vi "Save Orientation History.vi"() -> (2 "File Name refnum":refnum<file>, 3 "File Name path":path)   [LabVIEW 2016]
uses:
  navxmxp/roborio/labviewae/_TypeDefs/FRIC_navX_DeviceNumbersTypeDef.ctl
  <vilib>/Utility/file.llb/Write Delimited Spreadsheet (DBL).vi
panel:
  out "iterations":i32
  in  "Device Number":T1
  out "error out":errorcluster
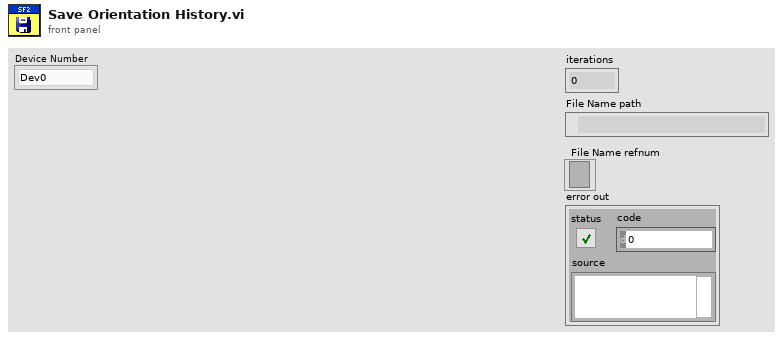
[diagram p1: front panel]
types:
  T1 = typedef "FRIC_navX_DeviceNumbersTypeDef.ctl" = enum16{"Dev0", "Dev1", "Dev2", "Dev3"}
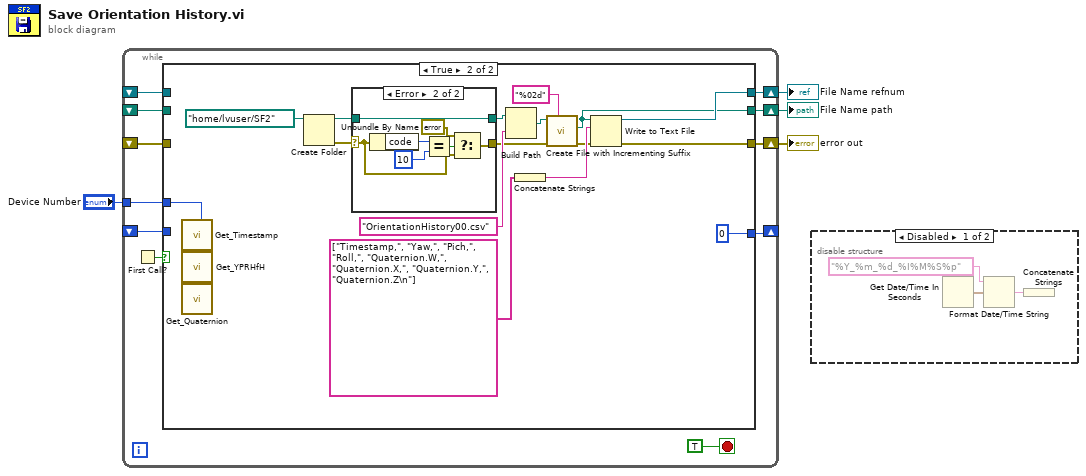
[diagram p0: block diagram]
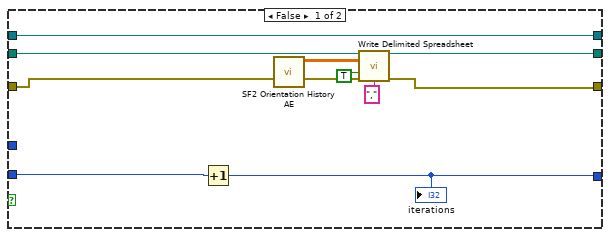
[diagram p3: hidden frame]
diagram:
  n1 = while {
    shift-right: [w15] -> w4
    shift-left: _ -> [w11]
    shift-right: [w14] -> w1
    shift-left: _ -> [w10]
    shift-right: [w9] -> w3
    shift-left: _ -> [w8]
    tunnel: "Device Number" -> [w7]
    shift-right: [w6] -> _
    shift-left: _ -> [w5]
    stop <- TRUE stop-if-true
    n2 = First Call?() -> (First Call?: T/F=w12:bool)
    n3 = case shown="True" w12 {
      tunnel: [w23 w38] -> w15
      tunnel: [w22 w37] -> w14
      tunnel: w11 -> [w23 _]
      tunnel: w10 -> [w21 _]
      tunnel: [w24 w26] -> w9
      tunnel: w8 -> [w25 _]
      tunnel: w7 -> [_ w33]
      tunnel: [w16 0] -> w6
      tunnel: w5 -> [w17 _]
      frame False {
        n4 = Increment(x=w17) -> (x+1=w16:i32)
        "iterations" <- w16
        n5 = call "SF2 Orientation History AE.vi"() -> ("SF2 Buffer (out)"=w18:dbl[][])  [unwired: 10 in, 1 out]
        n6 = call-poly <vilib>:"Write Delimited Spreadsheet.vi"("file path (dialog if empty)"=w25, "2D data"=w18, "append to file? (new file:F)"=TRUE, "error in (no error)"=w21, "delimiter (\\t)"="," ("delimiter (\\t)")) -> ("new file path (Not A Path if cancelled)"=w24:path, "error out"=w22:errorcluster)  [unwired: 9 in]
      }
      frame True {
        n7 = call "Get_Timestamp.vi"("Device Number"=w33) -> ()  [unwired: 10 in, 1 out]
        n8 = call "Get_YPRHfH.vi"("Device Number"=w33) -> ()  [unwired: 10 in, 1 out]
        n9 = call "Get_Quaternion.vi"("Device Number"=w33) -> ()  [unwired: 10 in, 1 out]
        n10 = Create Folder(path (use dialog)=path "/home/lvuser/SF2") -> (created path=w34:path, error out=w36:errorcluster)  [unwired: 2 in, 1 out]
        n11 = case shown="Error" w36 {
          selector: w36 -> [w42 w46]
          tunnel: w34 -> [w43 w50]
          tunnel: [w43 w50] -> w35
          tunnel: [w42 w45] -> w28
          frame No Error {
          }
          frame Error {
            n12 = Unbundle By Name(w46) -> ("code"=w49:i32)
            n13 = Equal?(x=w49, y=10) -> (x = y?=w44:bool)
            n14 = Select(t=errorcluster {"status"=FALSE, "code"=0, "source"=""} ("error IO"), s=w44, f=w46) -> (s? t:f=w45:errorcluster)
          }
        }
        n15 = Build Path(base path=w35, name or relative path="OrientationHistory00.csv") -> (appended path=w30:path)
        n16 = Concatenate Strings(string[] ["Timestamp,", "Yaw,", "Pich,", "Roll,", "Quaternion.W,", "Quaternion.X,", "Quaternion.Y,", "Quaternion.Z\n"]) -> (w39:string)
        n17 = call <vilib>:"Create File with Incrementing Suffix.vi"("format string (\" (%d)\")"="%02d" ("format string (\" (%d)\")"), "error in (no error)"=w28, "file path"=w30) -> ("error out"=w27:errorcluster, "actual path"=w26:path)  [unwired: 6 in, 1 out]
        n18 = Write to Text File(file (use dialog)=w26, text=w39, error in=w27) -> (refnum out=w38:refnum<file>, error out=w37:errorcluster)  [unwired: 1 in, 1 out]
      }
    }
  }
  "File Name refnum" <- w4
  "File Name path" <- w3
  "error out" <- w1
  n19 = disable-structure shown="Disabled" {
    frame Disabled {
      n20 = Get Date/Time In Seconds() -> (seconds since 1Jan1904=w52:timestamp)
      n21 = Format Date/Time String(time format string (%c)="%Y_%m_%d_%I%M%S%p", seconds (now)=w52) -> (date/time string=w51:string)  [unwired: 1 in]
      n22 = Concatenate Strings(w51) -> ()  [unwired: 1 out]
    }
    frame Enabled {
    }
  }
